vi "RichToFlatni_xnet_can_bm_api_Session.vi"(5 "OutputClusterType":T1, 11 "InputCluster":T2) -> (3 "OutputCluster":T1)   [LabVIEW 2025, in "xnet_can_bus_monitor_api_client.lvlib"]
uses:
  xnet_can_bus_monitor_api_client.lvlib
  ni_xnet_can_bm_api_Session.ctl
  ni_xnet_can_bm_api_Session_Flat.ctl
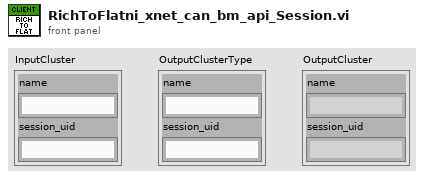
[diagram p1: front panel]
types:
  T1 = typedef "xnet_can_bus_monitor_api_client.lvlib/ni_xnet_can_bm_api_Session_Flat.ctl" = cluster{"name":string, "session_uid":string}
  T2 = typedef "xnet_can_bus_monitor_api_client.lvlib/ni_xnet_can_bm_api_Session.ctl" = cluster{"name":string, "session_uid":string}
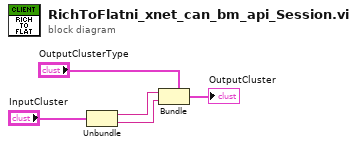
[diagram p0: block diagram]
diagram:
  n1 = Unbundle "Unbundle"("InputCluster") -> ("name"=w2:string, "session_uid"=w1:string)
  n2 = Bundle "Bundle"(cluster="OutputClusterType", "name"=w2, "session_uid"=w1) -> (→"OutputCluster":T1)
